vi "CmdexLedClr.vi"(8 "Uart Input":cluster{u64} {"?" format="%x"}, 10 "LED Id":enum16{"LED0", "LED1", "LED2", "LED3"}(ring), 11 "Error Input":errorcluster) -> (0 "Uart Output":cluster{u64} {"?" format="%x"}, 3 "Error Output":errorcluster)   [LabVIEW 2019]
doc: "<B>Cmdex</B>\nTurns the LED OFF."
uses:
  dll/LabViewUart.dll
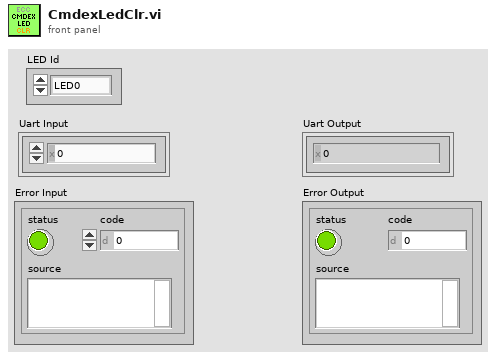
[diagram p1: front panel]
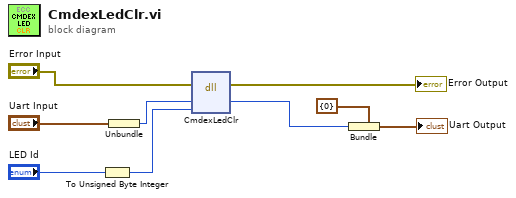
[diagram p0: block diagram]
diagram:
  n1 = To Unsigned Byte Integer(number="LED Id") -> (unsigned 8bit integer=w4:u8)
  n2 = Unbundle("Uart Input") -> (w6:u64)
  n3 = dll-call lib="D:/Google Drive/INC-2020/INC352/INC352-2020/LabVIEW/examples/uart-cmdex/SubVI/dll/LabViewUart.dll" fn="CmdexLedClr"(error in="Error Input", "Uart Handle"=w6, "id"=w4) -> (error out=→"Error Output":errorcluster, "Uart Handle"=w1:u64)  [unwired: 4 in, 1 out]
  n4 = Bundle(cluster=cluster{u64} {0}, w1) -> (→"Uart Output":cluster{u64})
